vi "array_to_Javascript_variable.vi"(7 "array":dbl[](array[numeric]), 10 "variable_name":string) -> (0 "variable_string":string)   [LabVIEW 2013]
doc: "Saves the xy graph to a javascript file usable by mjs_plot.js."
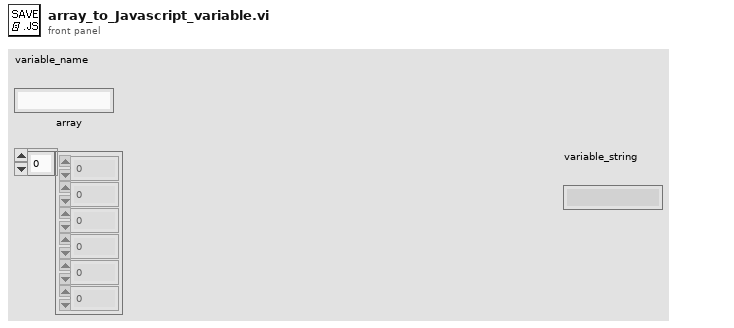
[diagram p1: front panel]
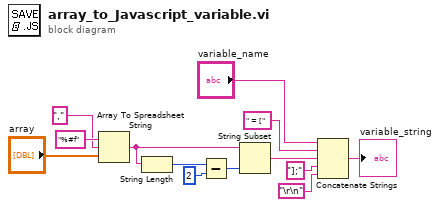
[diagram p0: block diagram]
diagram:
  n1 = Array To Spreadsheet String(delimiter (Tab)="," ("string"), array="array", 3:"%#f" ("format string")) -> (spreadsheet string=w7:string)
  n2 = String Length(string=w7) -> (length=w8:i32)
  n3 = Subtract(x=w8, y=2) -> (x-y=w9:i32)
  n4 = String Subset(string=w7, length (rest)=w9) -> (substring=w4:string)  [unwired: 1 in]
  n5 = Concatenate Strings("variable_name", " = [", w4, "];", "\r\n") -> (→"variable_string":string)
